vi "Create Queues.vi"(8 "Error In":errorcluster) -> (0 "Error Out":errorcluster)   [LabVIEW 2017]
uses:
  Message Cluster.ctl
  Reference Action.ctl
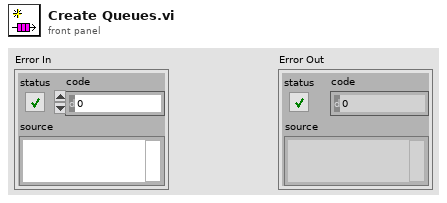
[diagram p1: front panel]
types:
  T1 = typedef "Reference Action.ctl" = enum16{"Set", "Get"}
  T2 = typedef "Message Cluster.ctl" = cluster{"Message":string, "Message Data":variant}
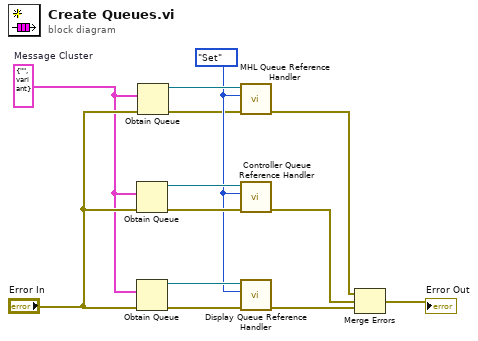
[diagram p0: block diagram]
diagram:
  w5 = Reference_Action."Set" ("Reference Action")
  w1 = T2 {"Message"="", "Message Data"=variant}  # Message Cluster
  n1 = Obtain Queue(element data type=w1, error in (no error)="Error In") -> (queue out=w8:refnum<queue>, error out=w13:errorcluster)  [unwired: 3 in, 1 out]
  n2 = Obtain Queue(element data type=w1, error in (no error)="Error In") -> (queue out=w7:refnum<queue>, error out=w12:errorcluster)  [unwired: 3 in, 1 out]
  n3 = Obtain Queue(element data type=w1, error in (no error)="Error In") -> (queue out=w6:refnum<queue>, error out=w2:errorcluster)  [unwired: 3 in, 1 out]
  n4 = call "MHL Queue Reference Handler.vi"("Error In"=w2, "Reference Action"=w5, "Queue Ref In"=w6) -> ("Error Out"=w3:errorcluster)  [unwired: 7 in, 1 out]
  n5 = call "Controller Queue Reference Handler.vi"("Error In"=w13, "Reference Action"=w5, "Queue Ref In"=w8) -> ("Error Out"=w10:errorcluster)  [unwired: 7 in, 1 out]
  n6 = call "Display Queue Reference Handler.vi"("Error In"=w12, "Reference Action"=w5, "Queue Ref In"=w7) -> ("Error Out"=w11:errorcluster)  [unwired: 7 in, 1 out]
  n7 = Merge Errors(w3, w10, w11) -> (→"Error Out":errorcluster)
